vi "Sequencer Main.vi"() -> ()   [LabVIEW 2018] (continued)
                                n1517 = global write "Global Variable.vi" "Retest ON"(TRUE ("Retest ON")) -> ()
                                }
                                }
                                }
                                frame True {
                                }
                              }
                            }
                          }
                        }
                        frame 42 {
                          # "BlueTooht Case\nEsp32 Reset"
                          # "Test ADB Bluetooth"
                          n1518 = Unbundle By Name(w2603) -> ("Parameters"=w2594:string, "Step Description"=w2591:string, "Test Values.Upper Limit"=w2598:dbl, "Test Values.Lower Limit"=w2597:dbl)  [unwired: 1 out]
                          n1519 = in-place {
                            in-place-border: w2594 -> [w2673]
                            in-place-border: [w2669] -> w2593
                            in-place-border: [w2668] -> w2592
                            # "Str \"fase\" exist"
                            n1520 = To Lower Case(string=w2673) -> (all lower case string=w2674:string)
                            n1521 = Match Pattern(string=w2674, regular expression="false") -> (after substring=w2671:string, offset past match=w2670:i32)  [unwired: 1 in, 2 out]
                            n1522 = Greater Or Equal To 0?(x=w2670) -> (x >= 0?=w2668:bool)
                            n1523 = case shown="True" w2668 {
                              tunnel: w2671 -> [_ w2677]
                              tunnel: [string[] [] w2676] -> w2669
                              frame False {
                                (unwired) ""
                              }
                              frame True {
                                n1524 = while {
                                shift-right: [w2681] -> _
                                shift-left: w2677 -> [w2682]
                                tunnel: [w2678] -> w2676 mode=indexing
                                stop <- w2680 stop-if-true
                                # "Get Array of Sub Parametrs"
                                n1525 = Match Pattern(string=w2682, regular expression=":") -> (before substring=w2678:string, after substring=w2681:string, offset past match=w2679:i32)  [unwired: 1 in, 1 out]
                                n1526 = Less Than 0?(x=w2679) -> (x < 0?=w2680:bool)
                                }
                              }
                            }
                          }
                          n1527 = property on="Msg Str" class="Str"("Value"=w2591) -> ()  [unwired: 2 in, 2 out]
                          n1528 = global read "Global Variable.vi" "COM Port BLE"() -> (w2588:refnum<visa-resource-name>)
                          n1529 = invoke on="Serial CMD Mon" class="Str" method="Reinit To Default"() -> (error out=w2587:errorcluster)  [unwired: 3 in, 2 out]
                          n1530 = property on="Tab Control Msg" class="TabCtl (strict)"("Value"=T4."Serial" ("Tab Control Msg")) -> (error out=w2601:errorcluster)  [unwired: 2 in, 1 out]
                          n1531 = flat-sequence {
                            tunnel: w2601 -> [w2611]
                            tunnel: w2598 -> [_]
                            tunnel: w2597 -> [_]
                            tunnel: w2594 -> [w2610]
                            tunnel: [w2612] -> w2596
                            tunnel: ["Reset ESP_32"] -> w2595
                            tunnel: w2591 -> [w2609]
                            tunnel: [w2604] -> w2590
                            tunnel: [w2608] -> w2589
                            tunnel: w2588 -> [w2607]
                            tunnel: w2587 -> [_]
                            tunnel: [w2632] -> w2599
                            tunnel: [w2638] -> w2602
                            tunnel: w2596 -> [w2638]
                            tunnel: w2595 -> [w2632]
                            tunnel: w2593 -> [w2637]
                            tunnel: w2592 -> [w2635]
                            tunnel: w2590 -> [w2631]
                            tunnel: w2589 -> [w2630]
                            frame #0 {
                              # "Step TEST Description"
                              # "Step TEST Result"
                              n1532 = in-place {
                                in-place-border: w2610 -> [w2619]
                                in-place-border: w2611 -> [_]
                                in-place-border: w2609 -> [w2617]
                                in-place-border: [w2616] -> w2604
                                in-place-border: [w2617] -> w2608
                                in-place-border: w2607 -> [w2618]
                                in-place-border: [w2615] -> w2605
                                # "ADB BLE Name"
                                n1533 = while {
                                shift-right: [w2627] -> _
                                shift-left: w2619 -> [w2628]
                                tunnel: [w2624] -> w2620 mode=indexing
                                stop <- w2626 stop-if-true
                                # "Get Array of Parametrs"
                                n1534 = Match Pattern(string=w2628, regular expression=">") -> (before substring=w2624:string, after substring=w2627:string, offset past match=w2625:i32)  [unwired: 1 in, 1 out]
                                n1535 = Less Than 0?(x=w2625) -> (x < 0?=w2626:bool)
                                }
                                n1536 = call "ADB-LMS_Esp32_Rst.vi"("COM BLE Esp32"=w2618) -> ("Stat"=w2615:bool, "CMD Monitor"=w2616:string)  [unwired: 9 in]
                                n1537 = Index Array(array=w2620, index #1=0 ("index"), index #2=1 ("index"), index #3=2 ("index")) -> ()  [unwired: 3 out]
                              }
                              n1538 = local write "Serial CMD Mon"(w2604) -> ()
                              n1539 = case shown="True" w2605 {
                                tunnel: [enum16{"Idle", "PASS", "FALSE"}."FALSE" ("Step Test Result") enum16{"Idle", "PASS", "FALSE"}."PASS" ("Step Test Result")] -> w2612
                                frame False {
                                }
                                frame True {
                                }
                              }
                            }
                            frame #1 {
                              # "Str \"fase\" Present"
                              n1540 = in-place {
                                in-place-border: w2630 -> [w2641]
                                in-place-border: w2631 -> [w2640]
                                in-place-border: w2632 -> [w2639]
                                n1541 = call "Log Add Msg.vi"("Result"=w2639, "Communication"=w2640, "Description"=w2641) -> ("Out Msg"=w2642:string)
                                n1542 = property on="LogMsg" class="Str"("Text.Scroll Position"=inf) -> ()  [unwired: 2 in, 2 out]
                                n1543 = invoke on="LogMsg" class="Str" method="Append String"("string"=w2642) -> ()  [unwired: 3 in, 4 out]
                              }
                              n1544 = in-place {
                                in-place-border: w2637 -> [w2667]
                                in-place-border: [w2661] -> w2634
                                in-place-border: [w2660] -> w2633
                                # "GoTo Test-nmb"
                                # "ReTest Cyckles"
                                n1545 = Index Array(array=w2667, index #1=0, index #2=1, index #3=2) -> (element #2=w2663:string, element #3=w2662:string)  [unwired: 1 out]
                                n1546 = Decimal String To Number(string=w2663) -> (number=w2661:i32)  [unwired: 2 in, 1 out]
                                n1547 = Decimal String To Number(string=w2662) -> (number=w2660:i32)  [unwired: 2 in, 1 out]
                              }
                              n1548 = local read "Debugging"() -> (w2636:bool)
                              n1549 = case shown="False" w2636 {
                                tunnel: w2635 -> [w2647 _]
                                tunnel: w2634 -> [w2645 _]
                                tunnel: w2633 -> [w2644 _]
                                frame False {
                                # "No Debug Mode"
                                n1550 = in-place {
                                in-place-border: [w2649] -> w2646
                                n1551 = global read "Global Variable.vi" "Retest Cnt"() -> (w2650:i16)
                                n1552 = Equal?(x=w2650, y=i16 0) -> (x = y?=w2649:bool)
                                }
                                n1553 = case shown="True" w2647 {
                                tunnel: w2646 -> [_ w2654]
                                tunnel: w2645 -> [_ w2652]
                                tunnel: w2644 -> [_ w2651]
                                frame False {
                                }
                                frame True {
                                # "String \"false\" Present"
                                n1554 = global write "Global Variable.vi" "Retest Step Nmb"(w2652) -> ()
                                n1555 = global write "Global Variable.vi" "Retest Nmb"(w2651) -> ()
                                n1556 = case shown="False" w2654 {
                                tunnel: w2651 -> [_ w2659]
                                frame False {
                                n1557 = global read "Global Variable.vi" "Retest Cnt"() -> (w2657:i16)
                                n1558 = Decrement(x=w2657) -> (x-1=w2656:i16)
                                n1559 = global write "Global Variable.vi" "Retest Cnt"(w2656) -> ()
                                n1560 = Wait (ms)(milliseconds to wait=u32 1000) -> ()  [unwired: 1 out]
                                }
                                frame True {
                                # "if(Retest-OFF & Cnt=0)"
                                n1561 = Decrement(x=w2659) -> (x-1=w2658:i32)
                                n1562 = global write "Global Variable.vi" "Retest Cnt"(w2658) -> ()
                                }
                                }
                                n1563 = global write "Global Variable.vi" "Retest ON"(TRUE ("Retest ON")) -> ()
                                }
                                }
                                }
                                frame True {
                                }
                              }
                            }
                          }
                        }
                        frame 43 {
                          w2700 = "------------------------" ("string")
                          w2699 = "\r\n"
                          # "Step TEST Result"
                          # "Step Result Msg"
                          # "Str with \"false\" goto parameters"
                          # "Str \"false\" Preset"
                          # "Cmd Case"
                          # "Cmd Case"
                          n1564 = Unbundle By Name(w2713) -> ("Parameters"=w2695:string, "Step Description"=w2684:string, "Test Values.Numeric Value"=w2689:dbl, "Test Values.Upper Limit"=w2688:dbl, "Test Values.Lower Limit"=w2687:dbl)
                          n1565 = in-place {
                            in-place-border: w2695 -> [w2745]
                            in-place-border: [w2744] -> w2694
                            in-place-border: [w2743] -> w2692
                            # "STr \"fase\" exist"
                            n1566 = To Lower Case(string=w2745) -> (all lower case string=w2746:string)
                            n1567 = Match Pattern(string=w2746, regular expression="false") -> (after substring=w2748:string, offset past match=w2749:i32)  [unwired: 1 in, 2 out]
                            n1568 = Greater Or Equal To 0?(x=w2749) -> (x >= 0?=w2743:bool)
                            n1569 = case shown="True" w2743 {
                              tunnel: w2748 -> [_ w2752]
                              tunnel: [string[] [] w2751] -> w2744
                              frame False {
                                (unwired) ""
                              }
                              frame True {
                                n1570 = while {
                                shift-right: [w2756] -> _
                                shift-left: w2752 -> [w2757]
                                tunnel: [w2753] -> w2751 mode=indexing
                                stop <- w2755 stop-if-true
                                # "Get Array of Sub Parametrs"
                                n1571 = Match Pattern(string=w2757, regular expression=":") -> (before substring=w2753:string, after substring=w2756:string, offset past match=w2754:i32)  [unwired: 1 in, 1 out]
                                n1572 = Less Than 0?(x=w2754) -> (x < 0?=w2755:bool)
                                }
                              }
                            }
                          }
                          n1573 = while {
                            shift-right: [w2762] -> _
                            shift-left: w2695 -> [w2763]
                            tunnel: [w2759] -> w2697 mode=indexing
                            stop <- w2761 stop-if-true
                            # "Get Array of Parametrs"
                            n1574 = Match Pattern(string=w2763, regular expression=">") -> (before substring=w2759:string, after substring=w2762:string, offset past match=w2760:i32)  [unwired: 1 in, 1 out]
                            n1575 = Less Than 0?(x=w2760) -> (x < 0?=w2761:bool)
                          }
                          n1576 = Concatenate Strings(w2684, w2699, w2700, w2700, w2700, w2699) -> (w2701:string)
                          n1577 = property on="Tab Control Msg" class="TabCtl (strict)"("Value"=T21."Serial" ("Tab Control Msg")) -> (error out=w2711:errorcluster)  [unwired: 2 in, 1 out]
                          n1578 = property on="Serial CMD Mon" class="Str"("Value"=w2701) -> ()  [unwired: 2 in, 2 out]
                          n1579 = Index Array(array=w2697, index=0) -> (element=w2709:string)
                          n1580 = Index Array(array=w2697, index=1) -> (element=w2707:string)
                          n1581 = Index Array(array=w2697, index=2) -> (element=w2704:string)
                          n1582 = Index Array(array=w2697, index=3) -> (element=w2702:string)
                          n1583 = Index Array(array=w2697, index=4) -> (element=w2696:string)
                          n1584 = case shown="\"getpid\"" w2709 {
                            tunnel: w2711 -> [_ _ _ _ _ _ _ _ _ _]
                            tunnel: [enum16{"Idle", "PASS", "FALSE"}."FALSE" ("Step Test Result") w2772 w2806 w2837 w2868 w2899 w2943 w2955 w2990 w3019] -> w2710
                            tunnel: w2707 -> [_ _ _ _ _ _ _ _ _ _]
                            tunnel: w2704 -> [_ _ _ _ _ _ _ _ _ _]
                            tunnel: w2702 -> [_ _ _ _ _ _ _ _ _ _]
                            tunnel: w2696 -> [_ _ _ _ _ _ _ _ _ _]
                            tunnel: ["" w2770 w2804 w2835 w2866 w2897 w2933 w2953 w2987 w3017] -> w2686
                            tunnel: w2689 -> [_ _ _ _ _ _ _ _ _ _]
                            tunnel: w2688 -> [_ _ _ _ _ _ w2939 _ _ _]
                            tunnel: w2687 -> [_ _ _ _ _ _ w2938 _ _ _]
                            tunnel: ["" w2769 w2803 w2834 w2865 w2896 w2933 w2952 w2989 w3016] -> w2685
                            frame "False", Default {
                              n1585 = One Button Dialog(message="!Sequencer File Err") -> ()  [unwired: 1 in, 1 out]
                            }
                            frame "status" {
                              # "Param"
                              # "Cmd"
                              n1586 = flat-sequence {
                                tunnel: [w2784] -> w2774
                                tunnel: [w2783] -> w2773
                                tunnel: [w2782] -> w2771
                                tunnel: w2774 -> [w2791]
                                tunnel: w2773 -> [w2792]
                                tunnel: [w2793] -> w2772
                                tunnel: w2771 -> [w2786]
                                tunnel: [w2789] -> w2770
                                tunnel: [w2786] -> w2769
                                frame #0 {
                                w2775 = u16 0 items=["None", "XON/XOFF", "RTS/CTS", "XON/XOFF & RTS/CTS", "DTR/DSR", "XON/XOFF & DTR/DSR"] ("flow control (0:none)")
                                n1587 = global read "Global Variable.vi" "COM Port BLE"() -> (w2781:refnum<visa-resource-name>)
                                n1588 = call "ADB-Serial_WrRd.vi"("flow control (0:none)"=w2775, "Tx Deay"=u16 1, "Timeout(Sec)"=3.0, "PassString"="Idle", "Command"="status?", "ComPort"=w2781) -> ("error out"=w2783:errorcluster, "PASS"=w2784:bool, "received"=w2782:string)  [unwired: 3 in]
                                n1589 = invoke on="Serial CMD Mon" class="Str" method="Append String"("string"=w2782) -> ()  [unwired: 3 in, 4 out]
                                n1590 = Wait (ms)(milliseconds to wait=u32 500) -> ()  [unwired: 1 out]
                                }
                                frame #1 {
                                n1591 = call <userlib>:"Multi-line String to Array__ogtk.vi"("string"=w2786) -> ("lines"=w2788:string[])
                                n1592 = Index Array(array=w2788, index=5) -> (element=w2785:string)
                                n1593 = global read "Global Variable.vi" "Array Errors"() -> (w2796:errorcluster[])
                                n1594 = case shown="False" w2791 {
                                tunnel: w2786 -> [_ _]
                                tunnel: [FALSE TRUE] -> w2790
                                tunnel: [w2797 w2799] -> w2789
                                tunnel: w2785 -> [w2797 w2799]
                                frame False {
                                }
                                frame True {
                                }
                                }
                                n1595 = Replace Array Subset(array=w2796, new element=w2792, index=3) -> (w2795:errorcluster[])
                                n1596 = global write "Global Variable.vi" "Array Errors"(w2795) -> ()
                                n1597 = case shown="True" w2790 {
                                tunnel: [enum16{"Idle", "PASS", "FALSE"}."FALSE" ("Step Test Result") enum16{"Idle", "PASS", "FALSE"}."PASS" ("Step Test Result")] -> w2793
                                frame False {
                                # "Step TEST Result"
                                }
                                frame True {
                                # "Step TEST Result"
                                }
                                }
                                }
                              }
                            }
                            frame "esp32_rst" {
                              # "Param"
                              # "Cmd"
                              n1598 = flat-sequence {
                                tunnel: [w2818] -> w2808
                                tunnel: [w2817] -> w2807
                                tunnel: [w2816] -> w2805
                                tunnel: w2808 -> [w2822]
                                tunnel: w2807 -> [w2823]
                                tunnel: [w2824] -> w2806
                                tunnel: w2805 -> [w2819]
                                tunnel: [w2820] -> w2804
                                tunnel: [w2819] -> w2803
                                frame #0 {
                                w2809 = u16 0 items=["None", "XON/XOFF", "RTS/CTS", "XON/XOFF & RTS/CTS", "DTR/DSR", "XON/XOFF & DTR/DSR"] ("flow control (0:none)")
                                n1599 = global read "Global Variable.vi" "COM Port BLE"() -> (w2815:refnum<visa-resource-name>)
                                n1600 = call "ADB-Serial_WrRd.vi"("flow control (0:none)"=w2809, "Tx Deay"=u16 1, "Timeout(Sec)"=5.0, "PassString"="Starting_Esp32", "Command"="esp32_rst", "ComPort"=w2815) -> ("error out"=w2817:errorcluster, "PASS"=w2818:bool, "received"=w2816:string)  [unwired: 3 in]
                                n1601 = invoke on="Serial CMD Mon" class="Str" method="Append String"("string"=w2816) -> ()  [unwired: 3 in, 4 out]
                                n1602 = Wait (ms)(milliseconds to wait=u32 500) -> ()  [unwired: 1 out]
                                }
                                frame #1 {
                                n1603 = case shown="False" w2822 {
                                tunnel: w2819 -> [_ _]
                                tunnel: [FALSE TRUE] -> w2821
                                tunnel: ["Esp32 Restart: Err" "Esp32 Restart: Ok"] -> w2820
                                frame False {
                                }
                                frame True {
                                }
                                }
                                n1604 = global read "Global Variable.vi" "Array Errors"() -> (w2827:errorcluster[])
                                n1605 = Replace Array Subset(array=w2827, new element=w2823, index=3) -> (w2826:errorcluster[])
                                n1606 = global write "Global Variable.vi" "Array Errors"(w2826) -> ()
                                n1607 = case shown="True" w2821 {
                                tunnel: [enum16{"Idle", "PASS", "FALSE"}."FALSE" ("Step Test Result") enum16{"Idle", "PASS", "FALSE"}."PASS" ("Step Test Result")] -> w2824
                                frame False {
                                # "Step TEST Result"
                                }
                                frame True {
                                # "Step TEST Result"
                                }
                                }
                                }
                              }
                            }
                            frame "disconnect" {
                              # "Param"
                              # "Cmd"
                              n1608 = flat-sequence {
                                tunnel: [w2849] -> w2839
                                tunnel: [w2848] -> w2838
                                tunnel: [w2847] -> w2836
                                tunnel: w2839 -> [w2853]
                                tunnel: w2838 -> [w2854]
                                tunnel: [w2855] -> w2837
                                tunnel: w2836 -> [w2850]
                                tunnel: [w2851] -> w2835
                                tunnel: [w2850] -> w2834
                                frame #0 {
                                w2840 = u16 0 items=["None", "XON/XOFF", "RTS/CTS", "XON/XOFF & RTS/CTS", "DTR/DSR", "XON/XOFF & DTR/DSR"] ("flow control (0:none)")
                                n1609 = global read "Global Variable.vi" "COM Port BLE"() -> (w2846:refnum<visa-resource-name>)
                                n1610 = call "ADB-Serial_WrRd.vi"("flow control (0:none)"=w2840, "Tx Deay"=u16 1, "Timeout(Sec)"=5.0, "PassString"="__DISCONNECT__", "Command"="disconnect", "ComPort"=w2846) -> ("error out"=w2848:errorcluster, "PASS"=w2849:bool, "received"=w2847:string)  [unwired: 3 in]
                                n1611 = invoke on="Serial CMD Mon" class="Str" method="Append String"("string"=w2847) -> ()  [unwired: 3 in, 4 out]
                                n1612 = Wait (ms)(milliseconds to wait=u32 500) -> ()  [unwired: 1 out]
                                }
                                frame #1 {
                                n1613 = case shown="True" w2853 {
                                tunnel: w2850 -> [_ _]
                                tunnel: [FALSE TRUE] -> w2852
                                tunnel: ["Esp32 Client Disconnect Err" "Esp32 Client Disconnect Ok"] -> w2851
                                frame False {
                                }
                                frame True {
                                }
                                }
                                n1614 = global read "Global Variable.vi" "Array Errors"() -> (w2858:errorcluster[])
                                n1615 = Replace Array Subset(array=w2858, new element=w2854, index=3) -> (w2857:errorcluster[])
                                n1616 = global write "Global Variable.vi" "Array Errors"(w2857) -> ()
                                n1617 = case shown="True" w2852 {
                                tunnel: [enum16{"Idle", "PASS", "FALSE"}."FALSE" ("Step Test Result") enum16{"Idle", "PASS", "FALSE"}."PASS" ("Step Test Result")] -> w2855
                                frame False {
                                # "Step TEST Result"
                                }
                                frame True {
                                # "Step TEST Result"
                                }
                                }
                                }
                              }
                            }
                            frame "scan" {
                              # "Param"
                              # "Cmd"
                              n1618 = flat-sequence {
                                tunnel: [w2880] -> w2870
                                tunnel: [w2879] -> w2869
                                tunnel: [w2878] -> w2867
                                tunnel: w2870 -> [w2884]
                                tunnel: w2869 -> [w2885]
                                tunnel: [w2886] -> w2868
                                tunnel: w2867 -> [w2881]
                                tunnel: [w2882] -> w2866
                                tunnel: [w2881] -> w2865
                                frame #0 {
                                w2871 = u16 0 items=["None", "XON/XOFF", "RTS/CTS", "XON/XOFF & RTS/CTS", "DTR/DSR", "XON/XOFF & DTR/DSR"] ("flow control (0:none)")
                                n1619 = global read "Global Variable.vi" "COM Port BLE"() -> (w2877:refnum<visa-resource-name>)
                                n1620 = call "ADB-Serial_WrRd.vi"("flow control (0:none)"=w2871, "Tx Deay"=u16 1, "Timeout(Sec)"=20.0, "PassString"="End", "Command"="scan", "ComPort"=w2877) -> ("error out"=w2879:errorcluster, "PASS"=w2880:bool, "received"=w2878:string)  [unwired: 3 in]
                                n1621 = invoke on="Serial CMD Mon" class="Str" method="Append String"("string"=w2878) -> ()  [unwired: 3 in, 4 out]
                                n1622 = Wait (ms)(milliseconds to wait=u32 500) -> ()  [unwired: 1 out]
                                }
                                frame #1 {
                                n1623 = global read "Global Variable.vi" "Array Errors"() -> (w2889:errorcluster[])
                                n1624 = case shown="False" w2884 {
                                tunnel: w2881 -> [_ _]
                                tunnel: [FALSE TRUE] -> w2883
                                tunnel: ["Scan Err" "Scan Ok"] -> w2882
                                frame False {
                                }
                                frame True {
                                }
                                }
                                n1625 = Replace Array Subset(array=w2889, new element=w2885, index=3) -> (w2888:errorcluster[])
                                n1626 = global write "Global Variable.vi" "Array Errors"(w2888) -> ()
                                n1627 = case shown="True" w2883 {
                                tunnel: [enum16{"Idle", "PASS", "FALSE"}."FALSE" ("Step Test Result") enum16{"Idle", "PASS", "FALSE"}."PASS" ("Step Test Result")] -> w2886
                                frame False {
                                # "Step TEST Result"
                                }
                                frame True {
                                # "Step TEST Result"
                                }
                                }
                                }
                              }
                            }
                            frame "connect" {
                              # "Param"
                              # "Cmd"
                              n1628 = flat-sequence {
                                tunnel: [w2916] -> w2901
                                tunnel: [w2915] -> w2900
                                tunnel: [w2914] -> w2898
                                tunnel: w2901 -> [w2920]
                                tunnel: w2900 -> [w2921]
                                tunnel: [w2922] -> w2899
                                tunnel: w2898 -> [w2917]
                                tunnel: [w2918] -> w2897
                                tunnel: [w2917] -> w2896
                                frame #0 {
                                w2905 = ">"
                                w2908 = u16 0 items=["None", "XON/XOFF", "RTS/CTS", "XON/XOFF & RTS/CTS", "DTR/DSR", "XON/XOFF & DTR/DSR"] ("flow control (0:none)")
                                n1629 = global read "Global Variable.vi" "Baccode MEM"() -> (w2904:string)
                                n1630 = Concatenate Strings("connect", w2905, "LEDLMS", w2905, w2904) -> (w2903:string)
                                n1631 = global read "Global Variable.vi" "COM Port BLE"() -> (w2913:refnum<visa-resource-name>)
                                n1632 = call "ADB-Serial_WrRd.vi"("flow control (0:none)"=w2908, "Tx Deay"=u16 1, "Timeout(Sec)"=20.0, "PassString"="PASS", "Command"=w2903, "ComPort"=w2913) -> ("error out"=w2915:errorcluster, "PASS"=w2916:bool, "received"=w2914:string)  [unwired: 3 in]
                                n1633 = global write "Global Variable.vi" "BLE Data"("") -> ()
                                n1634 = invoke on="Serial CMD Mon" class="Str" method="Append String"("string"=w2914) -> ()  [unwired: 3 in, 4 out]
                                n1635 = Wait (ms)(milliseconds to wait=u32 500) -> ()  [unwired: 1 out]
                                }
                                frame #1 {
                                n1636 = global read "Global Variable.vi" "Array Errors"() -> (w2925:errorcluster[])
                                n1637 = case shown="True" w2920 {
                                tunnel: w2917 -> [_ w2928]
                                tunnel: [FALSE TRUE] -> w2919
                                tunnel: ["Connect To LMS FALSE" "Connect To LMS PASS"] -> w2918
                                frame False {
                                }
                                frame True {
                                n1638 = global write "Global Variable.vi" "BLE Data"(w2928) -> ()
                                }
                                }
                                n1639 = Replace Array Subset(array=w2925, new element=w2921, index=3) -> (w2924:errorcluster[])
                                n1640 = global write "Global Variable.vi" "Array Errors"(w2924) -> ()
                                n1641 = case shown="True" w2919 {
                                tunnel: [enum16{"Idle", "PASS", "FALSE"}."FALSE" ("Step Test Result") enum16{"Idle", "PASS", "FALSE"}."PASS" ("Step Test Result")] -> w2922
                                frame False {
                                # "Step TEST Result"
                                }
                                frame True {
                                # "Step TEST Result"
                                }
                                }
                                }
                              }
                            }
                            frame "getrssi" {
                              w2935 = "rssi:"
                              # "Param"
                              # "Cmd"
                              n1642 = global read "Global Variable.vi" "BLE Data"() -> (w2942:string)
                              n1643 = Match Pattern(string=w2942, regular expression=w2935) -> (after substring=w2934:string, offset past match=w2941:i32)  [unwired: 1 in, 2 out]
                              n1644 = Greater Than 0?(x=w2941) -> (x > 0?=w2940:bool)
                              n1645 = case shown="True" w2940 {
                                tunnel: w2934 -> [_ w2949]
                                tunnel: [-999 w2947] -> w2937
                                frame False {
                                }
                                frame True {
                                n1646 = Scan From String(format string="%d", input string=w2949, default 1=-999 ("default value 1")) -> (error out=w2945:errorcluster, output 1=w2947:i32)  [unwired: 2 in, 2 out]
                                n1647 = call <userlib>:"Clear All Errors__ogtk.vi"("Error In"=w2945) -> ()  [unwired: 3 in, 1 out]
                                }
                              }
                              n1648 = Concatenate Strings(w2935, w2934) -> (w2933:string)
                              n1649 = In Range and Coerce(upper limit=w2939, x=w2937, lower limit=w2938) -> (In Range?=w2936:bool)  [unwired: 1 out]
                              n1650 = case shown="True" w2936 {
                                tunnel: [enum16{"Idle", "PASS", "FALSE"}."FALSE" ("Step Test Result") enum16{"Idle", "PASS", "FALSE"}."PASS" ("Step Test Result")] -> w2943
                                frame False {
                                # "Step TEST Result"
                                }
                                frame True {
                                # "Step TEST Result"
                                }
                              }
                            }
                            frame "open" {
                              # "Param"
                              # "Cmd"
                              n1651 = flat-sequence {
                                tunnel: [w2967] -> w2957
                                tunnel: [w2966] -> w2956
                                tunnel: [w2965] -> w2954
                                tunnel: w2957 -> [w2969]
                                tunnel: w2956 -> [w2976]
                                tunnel: [w2977] -> w2955
                                tunnel: w2954 -> [w2973]
                                tunnel: [w2974] -> w2953
                                tunnel: [w2973] -> w2952
                                frame #0 {
                                w2958 = u16 0 items=["None", "XON/XOFF", "RTS/CTS", "XON/XOFF & RTS/CTS", "DTR/DSR", "XON/XOFF & DTR/DSR"] ("flow control (0:none)")
                                n1652 = global read "Global Variable.vi" "COM Port BLE"() -> (w2964:refnum<visa-resource-name>)
                                n1653 = call "ADB-Serial_WrRd.vi"("flow control (0:none)"=w2958, "Tx Deay"=u16 1, "Timeout(Sec)"=2.0, "PassString"="Chuck(1)", "Command"="cmd>open", "ComPort"=w2964) -> ("error out"=w2966:errorcluster, "PASS"=w2967:bool, "received"=w2965:string)  [unwired: 3 in]
                                n1654 = invoke on="Serial CMD Mon" class="Str" method="Append String"("string"=w2965) -> ()  [unwired: 3 in, 4 out]
                                n1655 = Wait (ms)(milliseconds to wait=u32 500) -> ()  [unwired: 1 out]
                                }
                                frame #1 {
                                n1656 = Match Pattern(string=w2973, regular expression="Chuck(3)") -> (offset past match=w2971:i32)  [unwired: 1 in, 3 out]
                                n1657 = global read "Global Variable.vi" "Array Errors"() -> (w2980:errorcluster[])
                                n1658 = Greater Than 0?(x=w2971) -> (x > 0?=w2968:bool)
                                n1659 = Or(x=w2968, y=w2969) -> (x .or. y?=w2970:bool)
                                n1660 = Replace Array Subset(array=w2980, new element=w2976, index=3) -> (w2979:errorcluster[])
                                n1661 = case shown="True" w2970 {
                                tunnel: [FALSE TRUE] -> w2975
                                tunnel: ["BLE LMS Open: Err" ("line") "BLE LMS Open: Ok" ("line")] -> w2974
                                frame False {
                                }
                                frame True {
                                }
                                }
                                n1662 = global write "Global Variable.vi" "Array Errors"(w2979) -> ()
                                n1663 = case shown="True" w2975 {
                                tunnel: [enum16{"Idle", "PASS", "FALSE"}."FALSE" ("Step Test Result") enum16{"Idle", "PASS", "FALSE"}."PASS" ("Step Test Result")] -> w2977
                                frame False {
                                # "Step TEST Result"
                                }
                                frame True {
                                # "Step TEST Result"
                                }
                                }
                                }
                              }
                            }
                            frame "passwd" {
                              n1664 = flat-sequence {
                                tunnel: [w3002] -> w2992
                                tunnel: [w3001] -> w2991
                                tunnel: [w3000] -> w2988
                                tunnel: w2992 -> [w3005]
                                tunnel: w2991 -> [w3006]
                                tunnel: [w3007] -> w2990
                                tunnel: [w3004] -> w2989
                                tunnel: w2988 -> [w3004]
                                tunnel: [w3003] -> w2987
                                frame #0 {
                                w2993 = u16 0 items=["None", "XON/XOFF", "RTS/CTS", "XON/XOFF & RTS/CTS", "DTR/DSR", "XON/XOFF & DTR/DSR"] ("flow control (0:none)")
                                n1665 = global read "Global Variable.vi" "COM Port BLE"() -> (w2999:refnum<visa-resource-name>)
                                n1666 = call "ADB-Serial_WrRd.vi"("flow control (0:none)"=w2993, "Tx Deay"=u16 1, "Timeout(Sec)"=2.0, "PassString"="Chuck(3)", "Command"="cmd>passwd admin", "ComPort"=w2999) -> ("error out"=w3001:errorcluster, "PASS"=w3002:bool, "received"=w3000:string)  [unwired: 3 in]
                                n1667 = invoke on="Serial CMD Mon" class="Str" method="Append String"("string"=w3000) -> ()  [unwired: 3 in, 4 out]
                                n1668 = Wait (ms)(milliseconds to wait=u32 250) -> ()  [unwired: 1 out]
                                }
                                frame #1 {
                                n1669 = global read "Global Variable.vi" "Array Errors"() -> (w3010:errorcluster[])
                                n1670 = case shown="True" w3005 {
                                tunnel: [enum16{"Idle", "PASS", "FALSE"}."FALSE" ("Step Test Result") enum16{"Idle", "PASS", "FALSE"}."PASS" ("Step Test Result")] -> w3007
                                tunnel: ["Err" "BLE Passwd --> Admin"] -> w3003
                                frame False {
                                # "Step TEST Result"
                                }
                                frame True {
                                # "Step TEST Result"
                                }
                                }
                                n1671 = Replace Array Subset(array=w3010, new element=w3006, index=3) -> (w3009:errorcluster[])
                                n1672 = global write "Global Variable.vi" "Array Errors"(w3009) -> ()
                                }
                              }
                            }
                            frame "getpid" {
                              # "Param"
                              # "Cmd"
                              n1673 = flat-sequence {
                                tunnel: [w3033] -> w3021
                                tunnel: [w3032] -> w3020
                                tunnel: [w3031] -> w3018
                                tunnel: [w3031] -> w3016
                                tunnel: [w3025] -> w3015
                                tunnel: w3021 -> [w3034]
                                tunnel: w3020 -> [w3044]
                                tunnel: [w3045] -> w3019
                                tunnel: [w3039] -> w3017
                                tunnel: w3018 -> [w3042]
                                tunnel: w3015 -> [w3037]
                                frame #0 {
                                (unwired) "LEDLMS"
                                w3026 = u16 0 items=["None", "XON/XOFF", "RTS/CTS", "XON/XOFF & RTS/CTS", "DTR/DSR", "XON/XOFF & DTR/DSR"] ("flow control (0:none)")
                                n1674 = global read "Global Variable.vi" "Wr PID"() -> (w3025:string)
                                n1675 = global read "Global Variable.vi" "COM Port BLE"() -> (w3030:refnum<visa-resource-name>)
                                n1676 = Concatenate Strings("cmd", ">") -> (w3022:string)
                                n1677 = call "ADB-Serial_WrRd.vi"("flow control (0:none)"=w3026, "Tx Deay"=u16 1, "Timeout(Sec)"=3.0, "PassString"=w3025, "Command"=w3022, "ComPort"=w3030) -> ("error out"=w3032:errorcluster, "PASS"=w3033:bool, "received"=w3031:string)  [unwired: 3 in]
                                n1678 = invoke on="Serial CMD Mon" class="Str" method="Append String"("string"=w3031) -> ()  [unwired: 3 in, 4 out]
                                n1679 = Wait (ms)(milliseconds to wait=u32 250) -> ()  [unwired: 1 out]
                                }
                                frame #1 {
                                n1680 = in-place {
                                in-place-border: w3044 -> [w3052]
                                in-place-border: [w3052] -> w3043
                                in-place-border: [w3049] -> w3040
                                in-place-border: w3042 -> [w3051]
                                in-place-border: [w3049] -> w3038
                                n1681 = call <userlib>:"Multi-line String to Array__ogtk.vi"("string"=w3051) -> ("lines"=w3050:string[])
                                n1682 = for {
                                tunnel: [w3058] -> w3049
                                tunnel: w3050 -> [w3055] mode=indexing
                                stop <- w3053 stop-if-true
                                n1683 = Match Pattern(string=w3055, regular expression="PID:" ("search string/char (-)")) -> (after substring=w3056:string, offset past match=w3054:i32)  [unwired: 1 in, 2 out]
                                n1684 = Greater Than 0?(x=w3054) -> (x > 0?=w3053:bool)
                                n1685 = String Subset(string=w3056, offset (0)=1, length (rest)=13 ("length (rest)")) -> (substring=w3058:string)
                                }
                                n1686 = global write "Global Variable.vi" "Rd PID"(w3049) -> ()
                                }
                                n1687 = Equal?(x=w3038, y=w3037) -> (x = y?=w3035:bool)
                                n1688 = global read "Global Variable.vi" "Array Errors"() -> (w3048:errorcluster[])
                                n1689 = And(x=w3035, y=w3034) -> (x .and. y?=w3036:bool)
                                n1690 = case shown="False" w3036 {
                                tunnel: [enum16{"Idle", "PASS", "FALSE"}."FALSE" ("Step Test Result") enum16{"Idle", "PASS", "FALSE"}."PASS" ("Step Test Result")] -> w3045
                                frame False {
                                # "Step TEST Result"
                                }
                                frame True {
                                # "Step TEST Result"
                                }
                                }
                                n1691 = Replace Array Subset(array=w3048, new element=w3043, index=3) -> (w3047:errorcluster[])
                                n1692 = Concatenate Strings("BLE PID: " ("string"), w3040) -> (w3039:string)
                                n1693 = global write "Global Variable.vi" "Array Errors"(w3047) -> ()
                                }
                              }
                            }
                          }
                          n1694 = local read "Debugging"() -> (w2693:bool)
                          n1695 = in-place {
                            in-place-border: w2694 -> [w2737]
                            in-place-border: [w2736] -> w2690
                            in-place-border: [w2735] -> w2691
                            # "GoTo Test-nmb"
                            # "ReTest Cyckles"
                            n1696 = Index Array(array=w2737, index #1=0, index #2=1, index #3=2) -> (element #2=w2741:string, element #3=w2742:string)  [unwired: 1 out]
                            n1697 = Decimal String To Number(string=w2741) -> (number=w2736:i32)  [unwired: 2 in, 1 out]
                            n1698 = Decimal String To Number(string=w2742) -> (number=w2735:i32)  [unwired: 2 in, 1 out]
                          }
                          n1699 = case shown="False" w2693 {
                            tunnel: w2692 -> [w2722 _]
                            tunnel: w2690 -> [w2720 _]
                            tunnel: w2691 -> [w2719 _]
                            frame False {
                              # "No Debug Mode"
                              n1700 = in-place {
                                in-place-border: [w2724] -> w2721
                                n1701 = global read "Global Variable.vi" "Retest Cnt"() -> (w2725:i16)
                                n1702 = Equal?(x=w2725, y=i16 0) -> (x = y?=w2724:bool)
                              }
                              n1703 = case shown="True" w2722 {
                                tunnel: w2721 -> [_ w2729]
                                tunnel: w2720 -> [_ w2727]
                                tunnel: w2719 -> [_ w2726]
                                frame False {
                                }
                                frame True {
                                # "String \"false\" Present"
                                n1704 = global write "Global Variable.vi" "Retest Step Nmb"(w2727) -> ()
                                n1705 = global write "Global Variable.vi" "Retest Nmb"(w2726) -> ()
                                n1706 = case shown="False" w2729 {
                                tunnel: w2726 -> [_ w2734]
                                frame False {
                                n1707 = global read "Global Variable.vi" "Retest Cnt"() -> (w2732:i16)
                                n1708 = Decrement(x=w2732) -> (x-1=w2731:i16)
                                n1709 = global write "Global Variable.vi" "Retest Cnt"(w2731) -> ()
                                n1710 = Wait (ms)(milliseconds to wait=u32 1000) -> ()  [unwired: 1 out]
                                }
                                frame True {
                                # "if(Retest-OFF & Cnt=0)"
                                n1711 = Decrement(x=w2734) -> (x-1=w2733:i32)
                                n1712 = global write "Global Variable.vi" "Retest Cnt"(w2733) -> ()
                                }
                                }
                                n1713 = global write "Global Variable.vi" "Retest ON"(TRUE ("Retest ON")) -> ()
                                }
                              }
                            }
                            frame True {
                            }
                          }
                          n1714 = in-place {
                            in-place-border: w2684 -> [w2716]
                            in-place-border: w2685 -> [w2715]
                            in-place-border: w2686 -> [w2714]
                            n1715 = call "Log Add Msg.vi"("Result"=w2714, "Communication"=w2715, "Description"=w2716) -> ("Out Msg"=w2717:string)
                            n1716 = property on="LogMsg" class="Str"("Text.Scroll Position"=inf) -> ()  [unwired: 2 in, 2 out]
                            n1717 = invoke on="LogMsg" class="Str" method="Append String"("string"=w2717) -> ()  [unwired: 3 in, 4 out]
                          }
                        }
                        frame 45 {
                          # "Retest Cnt=0 ?"
                          # "RFID Case\nArduino"
                          # "Test ADB LMS RFID"
                          n1718 = Unbundle By Name(w3078) -> ("Test Values.Upper Limit"=w3072:dbl, "Test Values.Lower Limit"=w3073:dbl, "Parameters"=w3075:string)  [unwired: 2 out]
                          n1719 = property on="Tab Control Msg" class="TabCtl (strict)"("Value"=T4."Msg" ("Tab Control Msg")) -> (error out=w3076:errorcluster)  [unwired: 2 in, 1 out]
                          n1720 = in-place {
                            in-place-border: w3076 -> [_]
                            in-place-border: w3075 -> [w3119]
                            in-place-border: [w3111] -> w3074
                            in-place-border: w3073 -> [w3110]
                            in-place-border: w3072 -> [w3109]
                            in-place-border: [w3108] -> w3071
                            in-place-border: [w3106] -> w3070
                            # "COMPORT OPEN?"
                            n1721 = while {
                              shift-right: [w3421] -> _
                              shift-left: w3119 -> [w3422]
                              tunnel: [w3418] -> w3115 mode=indexing
                              stop <- w3420 stop-if-true
                              # "Get Array of Parametrs"
                              n1722 = Match Pattern(string=w3422, regular expression=">") -> (before substring=w3418:string, after substring=w3421:string, offset past match=w3419:i32)  [unwired: 1 in, 1 out]
                              n1723 = Less Than 0?(x=w3419) -> (x < 0?=w3420:bool)
                            }
                            n1724 = Index Array(array=w3115, index #1=0 ("index"), index #2=1 ("index"), index #3=2 ("index")) -> (element #1=w3107:string)  [unwired: 2 out]
                            n1725 = global read "Global Variable.vi" "COM Port RFID"() -> (w3114:refnum<visa-resource-name>)
                            n1726 = while {
                              shift-right: [w3123] -> _
                              shift-left: w3107 -> [w3124]
                              tunnel: [w3120] -> w3106 mode=indexing
                              stop <- w3122 stop-if-true
                              # "Get Array of Sub Parametrs"
                              n1727 = Match Pattern(string=w3124, regular expression=":") -> (before substring=w3120:string, after substring=w3123:string, offset past match=w3121:i32)  [unwired: 1 in, 1 out]
                              n1728 = Less Than 0?(x=w3121) -> (x < 0?=w3122:bool)
                            }
                            n1729 = Not Equal?(x=w3114, y="???") -> (x != y?=w3112:bool)
                            n1730 = case shown="True" w3112 {
                              tunnel: [FALSE w3136] -> w3111
                              tunnel: w3110 -> [_ w3138]
                              tunnel: w3109 -> [_ w3137]
                              tunnel: ["..." w3131] -> w3108
                              frame False {
                              }
                              frame True {
                                n1731 = flat-sequence {
                                tunnel: [w3162] -> w3134
                                tunnel: [w3158] -> w3128
                                tunnel: w3134 -> [w3189]
                                tunnel: [w3175] -> w3130
                                tunnel: [w3165] -> w3133
                                tunnel: [w3174] -> w3132
                                tunnel: w3128 -> [w3170]
                                frame #0 {
                                w3151 = "--------------------"
                                w3152 = "\r\n"
                                n1732 = case shown="True" FALSE {
                                frame False {
                                }
                                frame True {
                                n1733 = in-place {
                                # "Debug ONLY!"
                                n1734 = global write "Global Variable.vi" "Rd PID"("2119050000012") -> ()
                                }
                                }
                                }
                                n1735 = Concatenate Strings("Test ADB-LMS FRID", w3152, w3151, w3151, w3152, "Please WAIT  (Delay 10s)", w3152, w3151, w3151) -> (w3154:string)
                                n1736 = property on="Msg Str" class="Str"("Value"=w3154) -> ()  [unwired: 2 in, 2 out]
                                }
                                frame #1 {
                                n1737 = global read "Global Variable.vi" "COM Port RFID"() -> (w3157:refnum<visa-resource-name>)
                                n1738 = VISA Clear(VISA resource name=w3157) -> (VISA resource name out=w3161:refnum<visa-resource-name>, error out=w3160:errorcluster)  [unwired: 1 in]
                                n1739 = call "RFID Get ID.vi"("ComPort"=w3161) -> ("error out"=w3159:errorcluster, "received"=w3162:string)  [unwired: 9 in]
                                n1740 = invoke on="Msg Str" class="Str" method="Append String"("string"=w3162) -> ()  [unwired: 3 in, 4 out]
                                n1741 = Merge Errors(w3159, w3160) -> (w3158:errorcluster)
                                }
                                frame #2 {
                                w3184 = "\\[(.*)\\]" ("regular expression")
                                n1742 = call <userlib>:"Multi-line String to Array__ogtk.vi"("string"=w3189) -> ("lines"=w3188:string[])
                                n1743 = global read "Global Variable.vi" "Array Errors"() -> (w3173:errorcluster[])
                                n1744 = Index Array(array=w3188, index #1=1 ("index"), index #2=4 ("index")) -> (element #1=w3185:string, element #2=w3183:string)
                                n1745 = global read "Global Variable.vi" "Rd PID"() -> (w3168:string)
                                n1746 = xnode "Match Regular Expression"("input string"=w3183, "regular expression"=w3184) -> ("whole match"=w3179:string)  [unwired: 4 in, 4 out]
                                n1747 = xnode "Match Regular Expression"("input string"=w3185, "regular expression"=w3184) -> ("whole match"=w3181:string)  [unwired: 4 in, 4 out]
                                n1748 = Replace Array Subset(array=w3173, new element=w3170, index=7) -> (w3172:errorcluster[])
                                n1749 = global write "Global Variable.vi" "Array Errors"(w3172) -> ()
                                n1750 = String Subset(string=w3181, offset (0)=1, length (rest)=3 ("offset (0)")) -> (substring=w3169:string)
                                n1751 = String Subset(string=w3179, offset (0)=8, length (rest)=13 ("length (rest)")) -> (substring=w3165:string)
                                n1752 = Decimal String To Number(string=w3169) -> (number=w3174:i32)  [unwired: 2 in, 1 out]
                                n1753 = Concatenate Strings("rssi: ", w3169, "db Rd-PID: <", w3168, ">", "\r\n", "RFID-PID: " ("string"), w3165) -> (w3175:string)
                                }
                                }
